vi "Set Created Queues.vi"(10 "Created Queues":map{string, refnum<data-value>}(c390), 11 "Queue Mailbox in":refnum<class "Queue Mailbox.lvclass">) -> (3 "Queue Mailbox out":refnum<class "Queue Mailbox.lvclass">)   [LabVIEW 2021, in "jettl.lvlib" / "Queue Mailbox.lvlib" / "Queue Mailbox.lvclass"]
uses:
  Queue Mailbox.lvclass
  Msg Strategy/Msg Strategy.lvclass
  Queue Mailbox.lvclass/Queue Mailbox.ctl
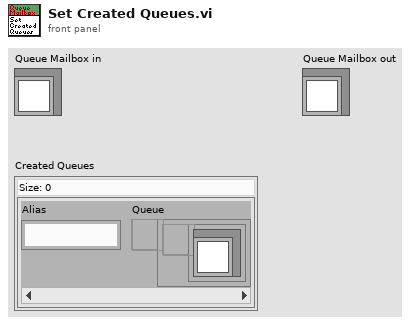
[diagram p1: front panel]
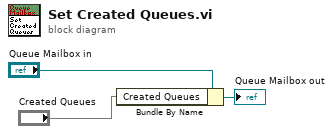
[diagram p0: block diagram]
diagram:
  n1 = Bundle By Name(cluster="Queue Mailbox in", "Created Queues"="Created Queues") -> (→"Queue Mailbox out":refnum<class "Queue Mailbox.lvclass">)
